vi "Read.vi"(8 "error in (no error)":errorcluster, 9 "Timeout":u32, 10 "Last message":refnum<class "BaseMessage.lvclass">, 11 "QueueReader in":refnum<class "QueueReader.lvclass">) -> (0 "error out":errorcluster, 1 "isAck?":bool, 2 "Responses":T1[](array[typedef]), 3 "QueueReader out":refnum<class "QueueReader.lvclass">)   [LabVIEW 2013, in "QueueReader.lvclass"]
doc: "Read a message from the remote destination"
uses:
  QueueReader.lvclass
  Message/BaseMessage/BaseMessage.lvclass
  response.ctl
  driver_status.ctl
  QueueReader.lvclass/QueueReader.ctl
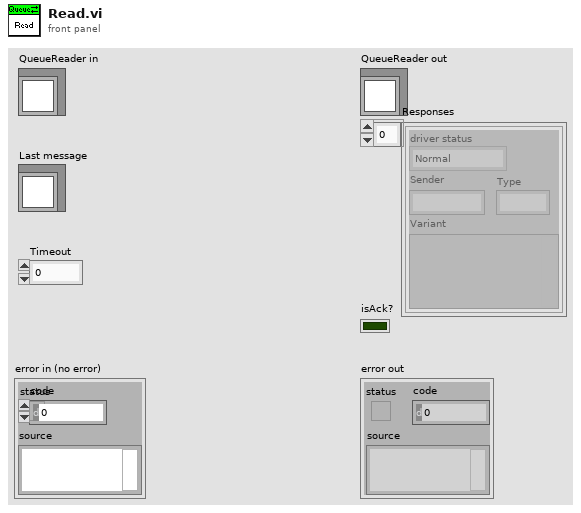
[diagram p1: front panel]
types:
  T1 = typedef "response.ctl" = cluster{"driver status":T2, "Sender":string, "Type":i32, "Variant":variant}
  T2 = typedef "driver_status.ctl" = enum16{"Normal", "Startup", "Connection lost", "Reconnected", "Timeout", "Idle", "Busy"}
  T3 = typedef "response queue.ctl" = refnum<queue>
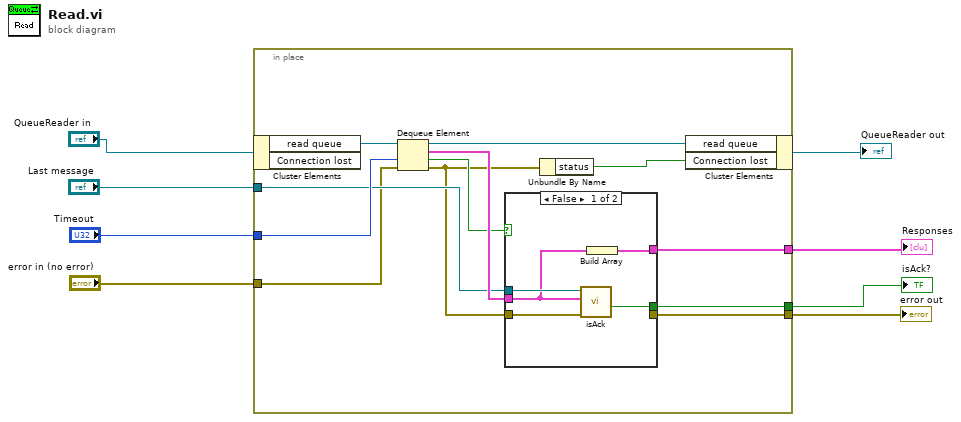
[diagram p0: block diagram]
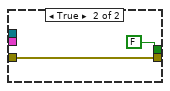
[diagram p2: hidden frame]
diagram:
  n1 = in-place "In Place Element Structure" {
    in-place-border: "Timeout" -> [w19]
    in-place-border: "Last message" -> [w17]
    in-place-border: [w16] -> w5
    in-place-border: "error in (no error)" -> [w15]
    in-place-border: [w14] -> w3
    in-place-border: [w12] -> w2
    n2 = in-place-cluster #1("QueueReader in") -> ("read queue"=w9:T3)  [unwired: 1 out]
    n3 = Dequeue Element(queue=w9, timeout in ms (-1)=w19, error in (no error)=w15) -> (queue out=w20:T3, element=w18:T1, timed out?=w13:bool, error out=w11:errorcluster)
    n4 = case shown="False" w13 {
      tunnel: w18 -> [w22 _]
      tunnel: w17 -> [w25 _]
      tunnel: [w24 FALSE ("isAck?")] -> w16
      tunnel: w11 -> [w23 w26]
      tunnel: [_ w26] -> w14
      tunnel: [w21 _] -> w12
      frame False {
        n5 = call-dynamic "isAck.vi"("error in (no error)"=w23, "response"=w22, "BaseMessage in"=w25) -> ("isAck?"=w24:bool)  [unwired: 6 in, 2 out]
        n6 = Build Array(w22) -> (w21:T1[])
      }
      frame True {
      }
    }
    n7 = Unbundle By Name(w11) -> ("status"=w10:bool)
    n8 = in-place-cluster #1("read queue"=w20, "Connection lost"=w10) -> (→"QueueReader out":refnum<class "QueueReader.lvclass">)
  }
  "error out" <- w3
  "Responses" <- w2
  "isAck?" <- w5
